vi "Convert Data to Chunks.vi"(7 "Chunk Size":i32, 9 "Chunk ID":u32, 11 "Data":string) -> (3 "Chunks":string[](array[string]))   [LabVIEW 2017]
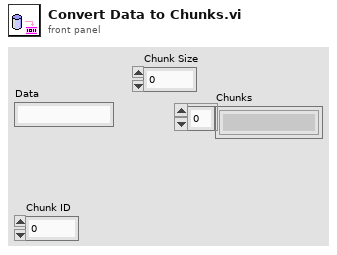
[diagram p1: front panel]
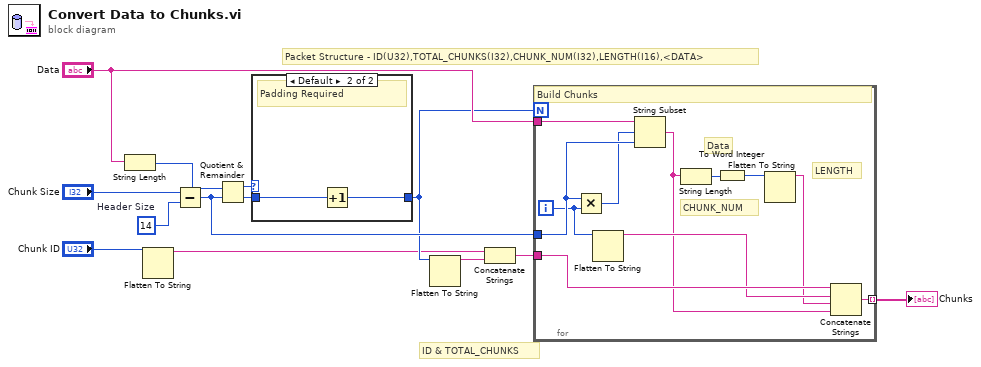
[diagram p0: block diagram]
diagram:
  w4 = 14  # Header Size
  # "ID & TOTAL_CHUNKS"
  # "Packet Structure - ID(U32),TOTAL_CHUNKS(I32),CHUNK_NUM(I32),LENGTH(I16),<DATA>"
  n1 = String Length(string="Data") -> (length=w1:i32)
  n2 = Flatten To String(anything="Chunk ID") -> (data string=w7:string)  [unwired: 3 in, 2 out]
  n3 = Subtract(x="Chunk Size", y=w4) -> (x-y=w11:i32)
  n4 = Quotient & Remainder(x=w1, y=w11) -> (x-y*floor(x/y)=w2:i32, floor(x/y)=w3:i32)
  n5 = case shown="Default" w2 {
    tunnel: w3 -> [w14 w16]
    tunnel: [w14 w15] -> w9
    frame 0 {
      # "Size Matches Chunk"
    }
    frame Default {
      # "Padding Required"
      n6 = Increment(x=w16) -> (x+1=w15:i32)
    }
  }
  n7 = Flatten To String(anything=w9) -> (data string=w8:string)  [unwired: 3 in, 2 out]
  n8 = Concatenate Strings(w7, w8) -> (w12:string)
  n9 = for {
    N: w9 -> [_]
    tunnel: "Data" -> [w27]
    tunnel: w11 -> [w26]
    tunnel: w12 -> [w22]
    tunnel: [w18] -> w13 mode=indexing
    i -> [w24]
    # "CHUNK_NUM"
    # "LENGTH"
    # "Data"
    # "Build Chunks"
    n10 = Multiply(x=w26, y=w24) -> (x*y=w25:i32)
    n11 = Flatten To String(anything=w24) -> (data string=w21:string)  [unwired: 3 in, 2 out]
    n12 = String Subset(string=w27, offset (0)=w25, length (rest)=w26) -> (substring=w19:string)
    n13 = String Length(string=w19) -> (length=w23:i32)
    n14 = To Word Integer(number=w23) -> (16bit integer=w17:i16)
    n15 = Flatten To String(anything=w17) -> (data string=w20:string)  [unwired: 3 in, 2 out]
    n16 = Concatenate Strings(w22, w21, w20, w19) -> (w18:string)
  }
  "Chunks" <- w13
